vi "Collapse.vi"(8 "error in (no error)":errorcluster, 11 "CollapsePanel in":refnum<class "CollapsePanel.lvclass">) -> (0 "error out":errorcluster, 3 "CollapsePanel out":refnum<class "CollapsePanel.lvclass">)   [LabVIEW 2021, in "CollapsePanel.lvclass"]
uses:
  CollapsePanel.lvclass
  CollapsePanel.lvclass/CollapsePanel.ctl
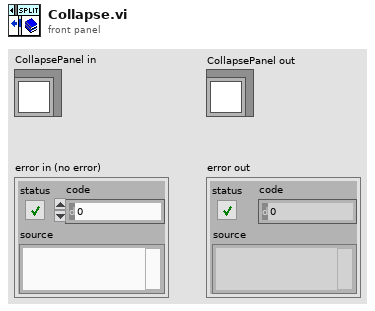
[diagram p1: front panel]
types:
  T1 = enum16{"No Scaling", "Scale All Objects", "Scale Single Object"}
  T2 = typedef "CollapsePanel.lvclass/collapse direction.ctl" = enum16{"Left", "Right", "Up", "Down"}
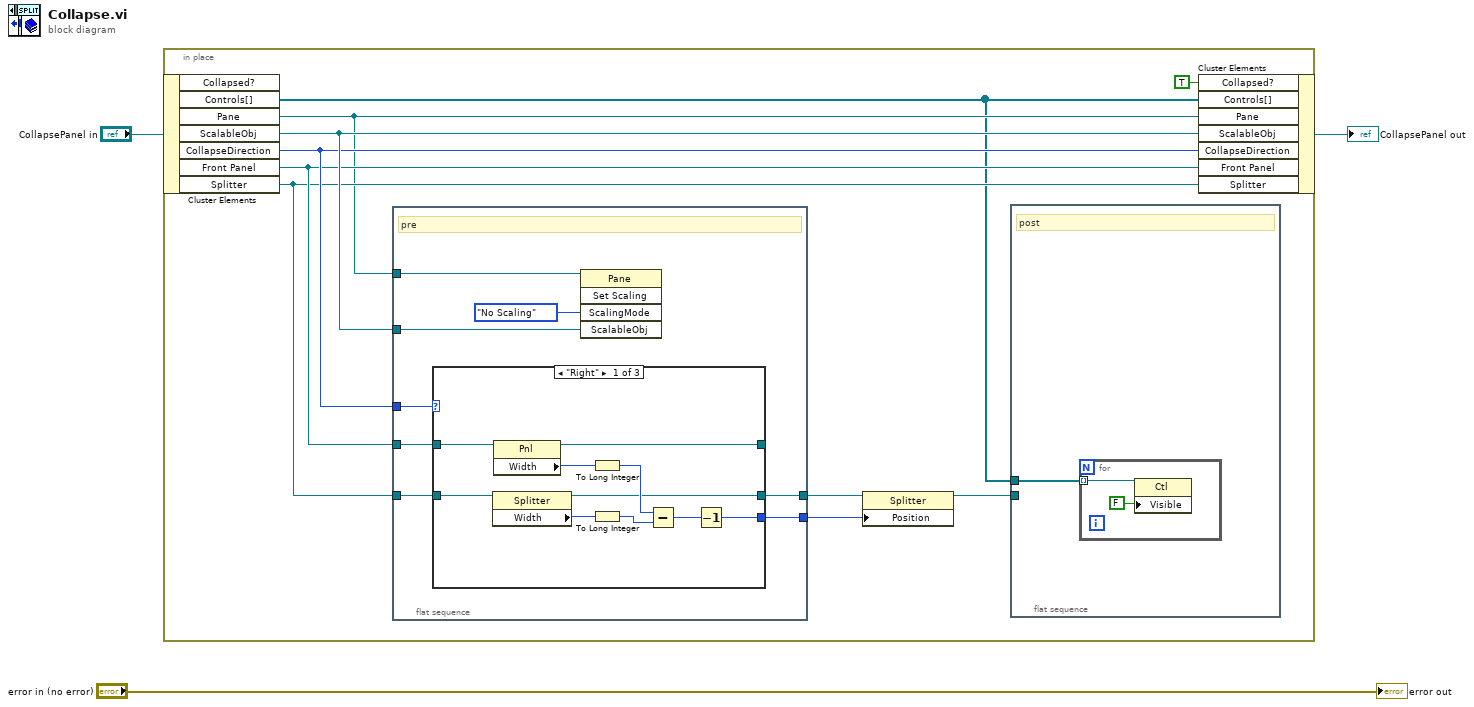
[diagram p0: block diagram]
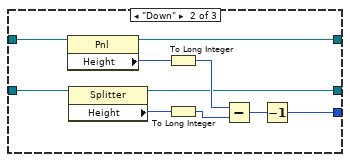
[diagram p2: hidden frame]
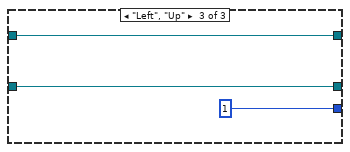
[diagram p3: hidden frame]
diagram:
  n1 = in-place {
    n2 = in-place-cluster #1("CollapsePanel in") -> ("Controls[]"=w7:refnum<vi>[], "Pane"=w8:refnum<vi>, "ScalableObj"=w12:refnum<vi>, "CollapseDirection"=w11:T2, "Front Panel"=w10:refnum<vi>, "Splitter"=w9:refnum<vi>)  [unwired: 1 out]
    n3 = flat-sequence {
      tunnel: [w23] -> w13
      tunnel: w12 -> [w22]
      tunnel: w11 -> [w21]
      tunnel: w10 -> [w20]
      tunnel: w9 -> [w19]
      tunnel: w8 -> [w18]
      tunnel: [w17] -> w6
      frame #0 {
        # "pre"
        n4 = case shown="\"Right\"" w21 {
          tunnel: w20 -> [w34 w44 w46]
          tunnel: w19 -> [w33 w43 w45]
          tunnel: [w27 w37 1] -> w23
          tunnel: [w26 w35 w46] -> _
          tunnel: [w25 w36 w45] -> w17
          frame "Right" {
            n5 = property class="Splitter"(reference=w33) -> (reference out=w25:refnum<vi>, "Width"=w31:u32)  [unwired: 1 in, 1 out]
            n6 = property class="Pnl"(reference=w34) -> (reference out=w26:refnum<vi>, "Width"=w32:u32)  [unwired: 1 in, 1 out]
            n7 = To Long Integer(number=w32) -> (32bit integer=w28:i32)
            n8 = To Long Integer(number=w31) -> (32bit integer=w29:i32)
            n9 = Subtract(x=w28, y=w29) -> (x-y=w30:i32)
            n10 = Decrement(x=w30) -> (x-1=w27:i32)
          }
          frame "Down" {
            n11 = property class="Pnl"(reference=w44) -> (reference out=w35:refnum<vi>, "Height"=w42:u32)  [unwired: 1 in, 1 out]
            n12 = property class="Splitter"(reference=w43) -> (reference out=w36:refnum<vi>, "Height"=w41:u32)  [unwired: 1 in, 1 out]
            n13 = To Long Integer(number=w42) -> (32bit integer=w38:i32)
            n14 = To Long Integer(number=w41) -> (32bit integer=w39:i32)
            n15 = Subtract(x=w38, y=w39) -> (x-y=w40:i32)
            n16 = Decrement(x=w40) -> (x-1=w37:i32)
          }
          frame "Left", "Up" {
          }
        }
        n17 = invoke class="Pane" method="Set Scaling"(reference=w18, "ScalingMode"=T1."No Scaling" ("Scaling Mode"), "ScalableObj"=w22) -> ()  [unwired: 2 in, 5 out]
      }
    }
    n18 = property class="Splitter"(reference=w6, "Position"=w13) -> (reference out=w5:refnum<vi>)  [unwired: 1 in, 1 out]
    n19 = flat-sequence {
      tunnel: w7 -> [w14]
      tunnel: w5 -> [_]
      frame #0 {
        # "post"
        n20 = for {
          tunnel: w14 -> [w15] mode=indexing
          n21 = property on="Property Node" class="Ctl"(reference=w15, "Visible"=FALSE) -> ()  [unwired: 1 in, 2 out]
        }
      }
    }
    n22 = in-place-cluster #1("Collapsed?"=TRUE, "Controls[]"=w7, "Pane"=w8, "ScalableObj"=w12, "CollapseDirection"=w11, "Front Panel"=w10, "Splitter"=w9) -> (→"CollapsePanel out":refnum<class "CollapsePanel.lvclass">)
  }
  "error out" <- "error in (no error)"
